vi "Full_D-mode.vi"(2 "Timeout (ms) 입력":i32, 3 "TCP 네트워크 연결 입력":refnum<k5>) -> (1 "TCP 네트워크 연결 출력":refnum<k5>)   [LabVIEW 2016]
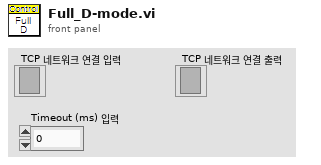
[diagram p1: front panel]
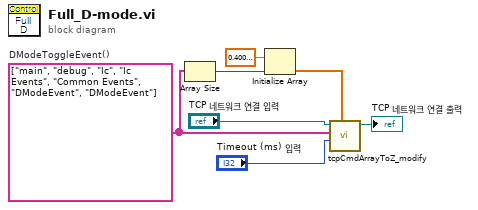
[diagram p0: block diagram]
diagram:
  w1 = string[] ["main", "debug", "Ic", "Ic Events", "Common Events", "DModeEvent", "DModeEvent"]  # DModeToggleEvent()
  n1 = Array Size(array=w1) -> (size(s)=w4:i32)
  n2 = Initialize Array(sgl 0.4 ("element"), w4) -> (w2:sgl[])
  n3 = call "tcpCmdArrayToZ_modify.vi"("Delay (sec)"=w2, "Timeout (ms)"="Timeout (ms) 입력", "Command array"=w1, "connection ID in"="TCP 네트워크 연결 입력") -> ("connection ID out"=→"TCP 네트워크 연결 출력":refnum<k5>)  [unwired: 3 in, 4 out]
